vi "Teleop.vi"(10 "Match Info":T2={"Autonomous Elapsed Seconds"=0.0, "TeleOp Elapsed Seconds"=0.0, "Disabled Elapsed Seconds"=0.0, "Visited Autonomous"=FALSE, "Visited TeleOp"=FALSE, "Visited Disabled"=FALSE, "Autonomous Settings"={"Autonomous Style"=enum."Independent", "VI Refnum"=refnum}}, 11 "Call Context":T3) -> ()   [LabVIEW 2019]
doc: "This VI is called for each enabled TeleOp packet received from the DS. It is typically used to read from joysticks and other inputs and update I/O or setpoints for timed control loops. It should complete and return within 20 milliseconds or risk missing DS packets."
uses:
  <vilib>/Rock Robotics/WPI/DriverStation/WPI_DriverStationDerivedRobotMode.ctl
  <vilib>/Rock Robotics/WPI/DriverStation/WPI_DriverStationMatch Info.ctl
  <vilib>/Rock Robotics/WPI/Utilities/WPI_GetSetVariantRefNum.vi
  <vilib>/Rock Robotics/Network Tables/NT Write Boolean Array.vi
  <vilib>/Rock Robotics/Network Tables/NT Write Numeric Array.vi
panel:
  in  "Enum":T1(ring)=enum."Two Controller Tank"
  in  "Controller 2 inverted":bool
  in  "Controller 2 Joystick":dbl min=0.0 max=6.0 step=1.0
  in  "Quickturn button":dbl min=0.0 max=12.0 step=1.0
  in  "Inverted One":bool
  in  "Inverted Two":bool
  in  "Joystick Two":dbl min=0.0 max=6.0 step=1.0
  in  "Joystick One":dbl min=0.0 max=6.0 step=1.0
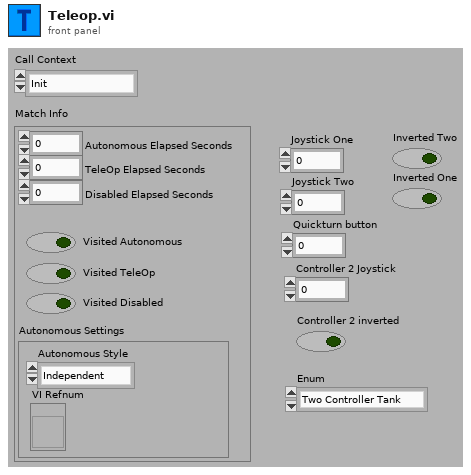
[diagram p1: front panel]
types:
  T1 = enum16{"Arcade", "One Controller Tank", "Two Controller Tank", "Cheesy Drive"}
  T2 = typedef "WPI_DriverStationMatch Info.ctl" = cluster{"Autonomous Elapsed Seconds":dbl, "TeleOp Elapsed Seconds":dbl, "Disabled Elapsed Seconds":dbl, "Visited Autonomous":bool, "Visited TeleOp":bool, "Visited Disabled":bool, "Autonomous Settings":cluster{"Autonomous Style":enum16{"Iterative", "Independent"}, "VI Refnum":refnum<vi>}}
  T3 = typedef "WPI_DriverStationDerivedRobotMode.ctl" = enum16{"Init", "Execute", "Stop"}
  T4 = enum16{"Arcade", "One Joystick Tank", "Two Joystick Tank", "Cheesy Drive", ""}
  T5 = typedef "WPI_JoystickDevRef.ctl" = cluster{"Device":T6}
  T6 = typedef "WPI_JoystickDeviceEnum.ctl" = enum16{"USB 0", "USB 1", "USB 2", "USB 3", "USB 4", "USB 5"}
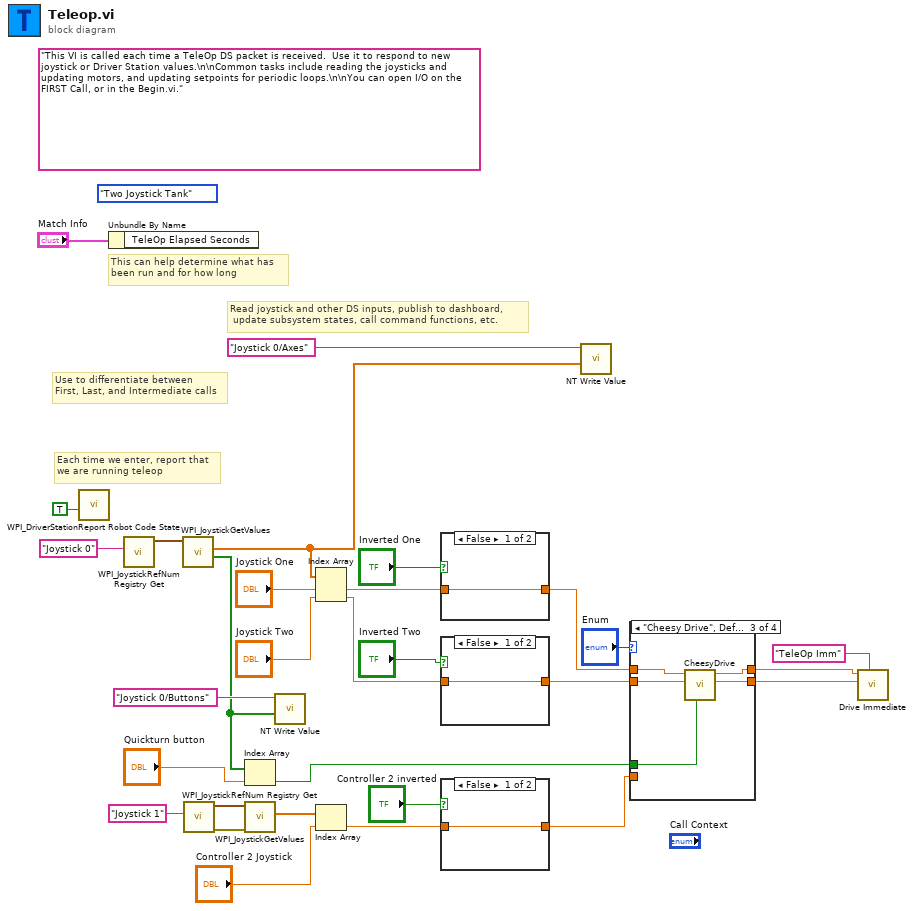
[diagram p0: block diagram]
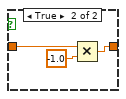
[diagram p2: hidden frame]
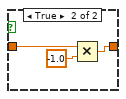
[diagram p3: hidden frame]
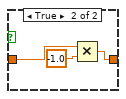
[diagram p4: hidden frame]
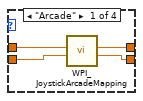
[diagram p5: hidden frame]
diagram:
  (unwired) T4."Two Joystick Tank"
  (unwired) "This VI is called each time a TeleOp DS packet is received.  Use it to respond to new joystick or Driver Station values.\n\nCommon tasks include reading the joysticks and updating motors, and updating setpoints for periodic loops.\n\nYou can open I/O on the FIRST Call, or in the Begin.vi."
  # "Read joystick and other DS inputs, publish to dashboard,\n update subsystem states, call command functions, etc."
  # "Each time we enter, report that\nwe are running teleop"
  # "Use to differentiate between\nFirst, Last, and Intermediate calls"
  # "This can help determine what has\nbeen run and for how long"
  n1 = call <vilib>:"WPI_DriverStationReport Robot Code State.vi"("TeleOp"=TRUE ("Autonomous")) -> ()  [unwired: 10 in, 1 out]
  n2 = Unbundle By Name("Match Info") -> ()  [unwired: 1 out]
  n3 = call <vilib>:"WPI_JoystickRefNum Registry Get.vi"("refnum name"="Joystick 0") -> ("JoystickDevRef"=w27:T5)  [unwired: 1 in, 9 out]
  n4 = call <vilib>:"WPI_JoystickGetValues.vi"("JoystickDevRef"=w27) -> ("Buttons"=w3:bool[], "Axes"=w24:dbl[])  [unwired: 6 in, 3 out]
  n5 = call <vilib>:"WPI_JoystickRefNum Registry Get.vi"("refnum name"="Joystick 1") -> ("error out"=w10:errorcluster, "JoystickDevRef"=w11:T5)  [unwired: 1 in, 8 out]
  n6 = Index Array(array=w3, index="Quickturn button") -> (element=w1:bool)
  n7 = call <vilib>:"WPI_JoystickGetValues.vi"("error in (no error)"=w10, "JoystickDevRef"=w11) -> ("Axes"=w8:dbl[])  [unwired: 5 in, 4 out]
  n8 = call-poly <vilib>:"NT Write Value.vi"("Boolean Array"=w3, "Name"="Joystick 0/Buttons") -> ()  [unwired: 9 in, 1 out]
  n9 = Index Array(array=w24, index #1="Joystick One", index #2="Joystick Two") -> (element #1=w18:dbl, element #2=w16:dbl)
  n10 = Index Array(array=w8, index="Controller 2 Joystick") -> (element=w5:dbl)
  n11 = case shown="False" "Inverted One" {
    tunnel: w18 -> [w31 w33]
    tunnel: [w31 w32] -> w17
    frame False {
    }
    frame True {
      n12 = Multiply(x=w33, y=-1.0) -> (x*y=w32:dbl)
    }
  }
  n13 = case shown="False" "Inverted Two" {
    tunnel: w16 -> [w35 w37]
    tunnel: [w35 w36] -> w15
    frame False {
    }
    frame True {
      n14 = Multiply(x=w37, y=-1.0) -> (x*y=w36:dbl)
    }
  }
  n15 = case shown="False" "Controller 2 inverted" {
    tunnel: w5 -> [w39 w41]
    tunnel: [w39 w40] -> w4
    frame False {
    }
    frame True {
      n16 = Multiply(x=w41, y=-1.0) -> (x*y=w40:dbl)
    }
  }
  n17 = call-poly <vilib>:"NT Write Value.vi"("Numeric Array"=w24, "Name"="Joystick 0/Axes") -> ()  [unwired: 9 in, 1 out]
  n18 = case shown="\"Cheesy Drive\", Default" "Enum" {
    tunnel: w17 -> [w46 w48 w53 w55]
    tunnel: w15 -> [w45 _ w52 w54]
    tunnel: [w44 w48 w50 w55] -> w14
    tunnel: [w43 w47 w49 w54] -> w13
    tunnel: w4 -> [_ w47 _ _]
    tunnel: w1 -> [_ _ w51 _]
    frame "Arcade" {
      n19 = call <vilib>:"WPI_JoystickArcadeMapping.vi"("Y axis value"=w45, "X axis value"=w46) -> ("Right Motor Value"=w43:dbl, "Left Motor Value"=w44:dbl)  [unwired: 8 in]
    }
    frame "Two Controller Tank" {
    }
    frame "Cheesy Drive", Default {
      n20 = call "CheesyDrive.vi"("Quickturn"=w51, "Wheel"=w52, "Throttle"=w53) -> ("Right PWM"=w49:dbl, "Left PWM"=w50:dbl)  [unwired: 7 in]
    }
    frame "One Controller Tank" {
    }
  }
  n21 = call "Drive Immediate.vi"("Description"="TeleOp Imm", "Right Setpoint"=w13, "Left Setpoint"=w14) -> ()  [unwired: 8 in, 1 out]
